vi "messaging_processor.vi"(2 "params":T1={"hla_adapter_port"=2222, "hla_adapter_ip"="", "listener_port"=2222}, 4 "is_simulation_mode":bool=TRUE) -> ()   [LabVIEW 2016]
uses:
  controls/messaging_processor_params.ctl
  controls/messaging_processor_actions.ctl
  controls/terminal_display_handler_actions.ctl
  controls/queue_assistant_actions.ctl
  controls/queue_type.ctl
  controls/event_assistant_actions.ctl
  controls/user_event_item.ctl
  controls/user_events.ctl
panel:
  in  "stop":bool
  in  "reset":bool
  in  "classpaths":string[](array[string])
  in  "exit":bool
  out "out_conn":bool
  out "in_conn":bool
  out "to_hla_history":string
  out "from_hla_history":string
  out "error out":errorcluster
  in  "error in (no error)":errorcluster
  # "Incoming From HLA"
  # "Outgoing To HLA"
  # "connected"
  # "connected"
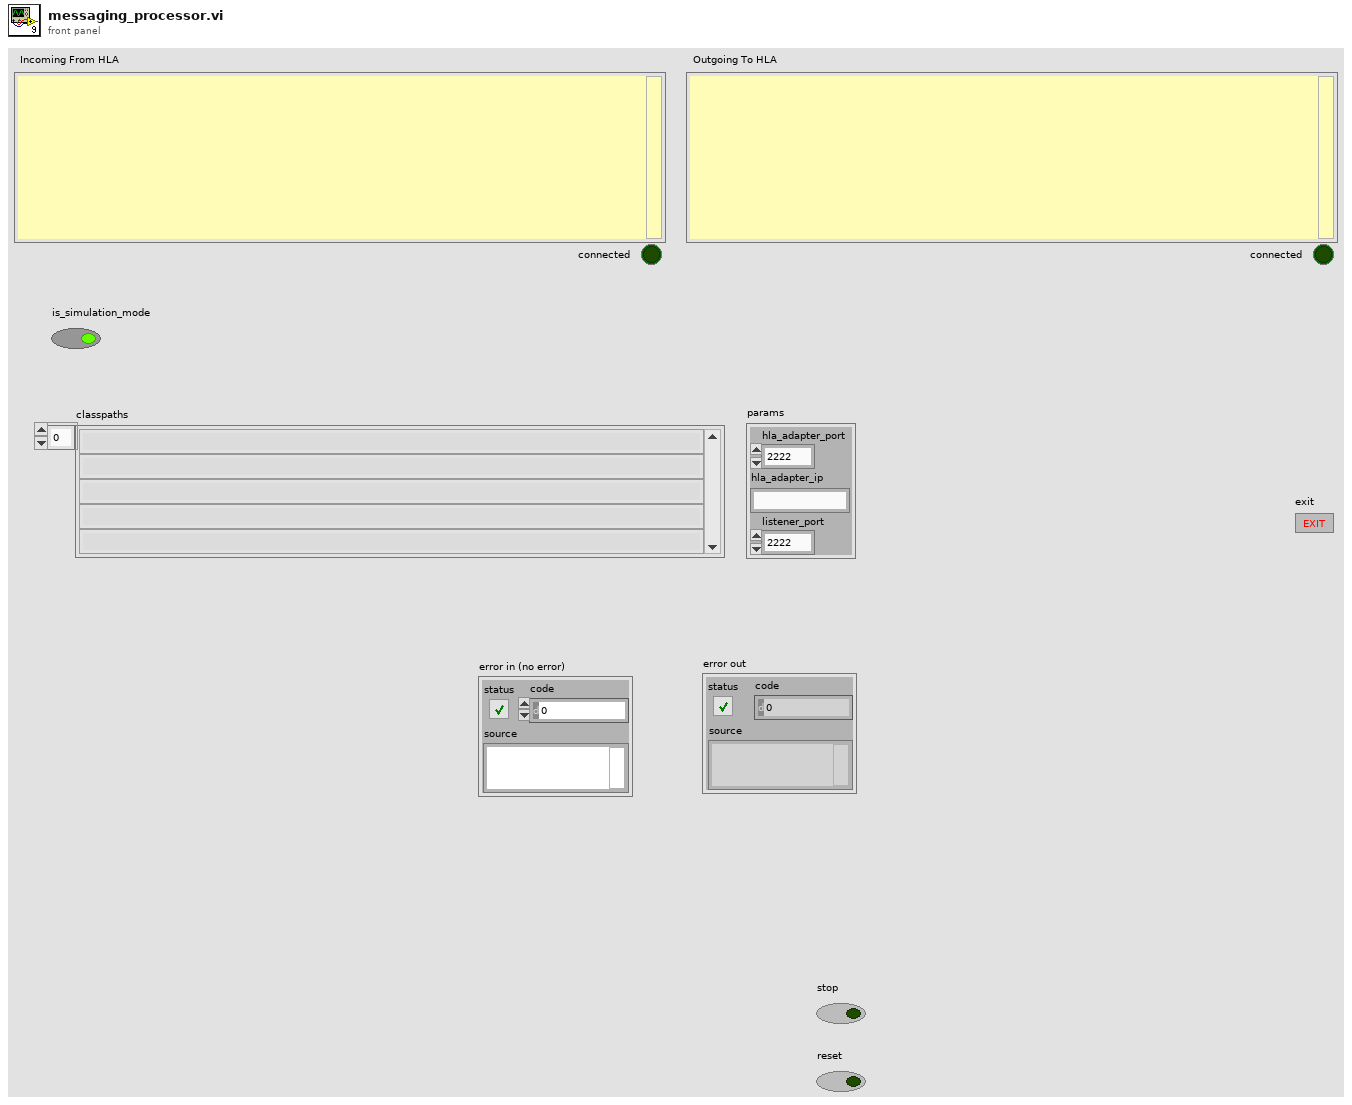
[diagram p1: front panel]
types:
  T1 = typedef "messaging_processor_params.ctl" = cluster{"hla_adapter_port":u16, "hla_adapter_ip":string, "listener_port":u16}
  T2 = typedef "messaging_processor_actions.ctl" = enum16{"-------- unused --------", "establish_connections", "exit", "init", "init_ui", "process_events"}
  T3 = typedef "terminal_display_handler_actions.ctl" = enum16{"clear", "clear_all", "init", "reset", "write"}
  T4 = typedef "queue_assistant_actions.ctl" = enum16{"--- unused ---", "bulk_enq_ahead", "bulk_enq_behind", "destroy", "empty?", "enq_ahead", "enq_behind", "flush", "get_queues", "init"}
  T5 = typedef "queue_references.ctl" = cluster{"entities_in":refnum<queue>, "entities_out":refnum<queue>, "timestep":refnum<queue>, "response":refnum<queue>}
  T6 = typedef "response.ctl" = cluster{"respType":T7, "flattenedContent":string}
  T7 = typedef "response_type.ctl" = string
  T8 = enum16{"Standard", "Buffered", "CRLF", "Immediate"}
  T9 = typedef "queue_type.ctl" = enum16{"all", "dostep", "entities_incoming", "entities_outoing", "response"}
  T10 = typedef "user_event_item.ctl" = cluster{"event":T11, "data":variant}
  T11 = typedef "user_events.ctl" = enum16{"abort", "do-step", "sim-end"}
  T12 = typedef "event_assistant_actions.ctl" = enum16{"--- unused ---", "destroy", "fire", "get_ref", "init"}
  T13 = typedef "lineitem_types.ctl" = enum16{"<unknown>", "received.dostep", "received.item", "received.simend"}
  T14 = typedef "entity.ctl" = cluster{"type":T15, "classPath":string, "params":string[][], "instanceName":string}
  T15 = typedef "entity_type.ctl" = string
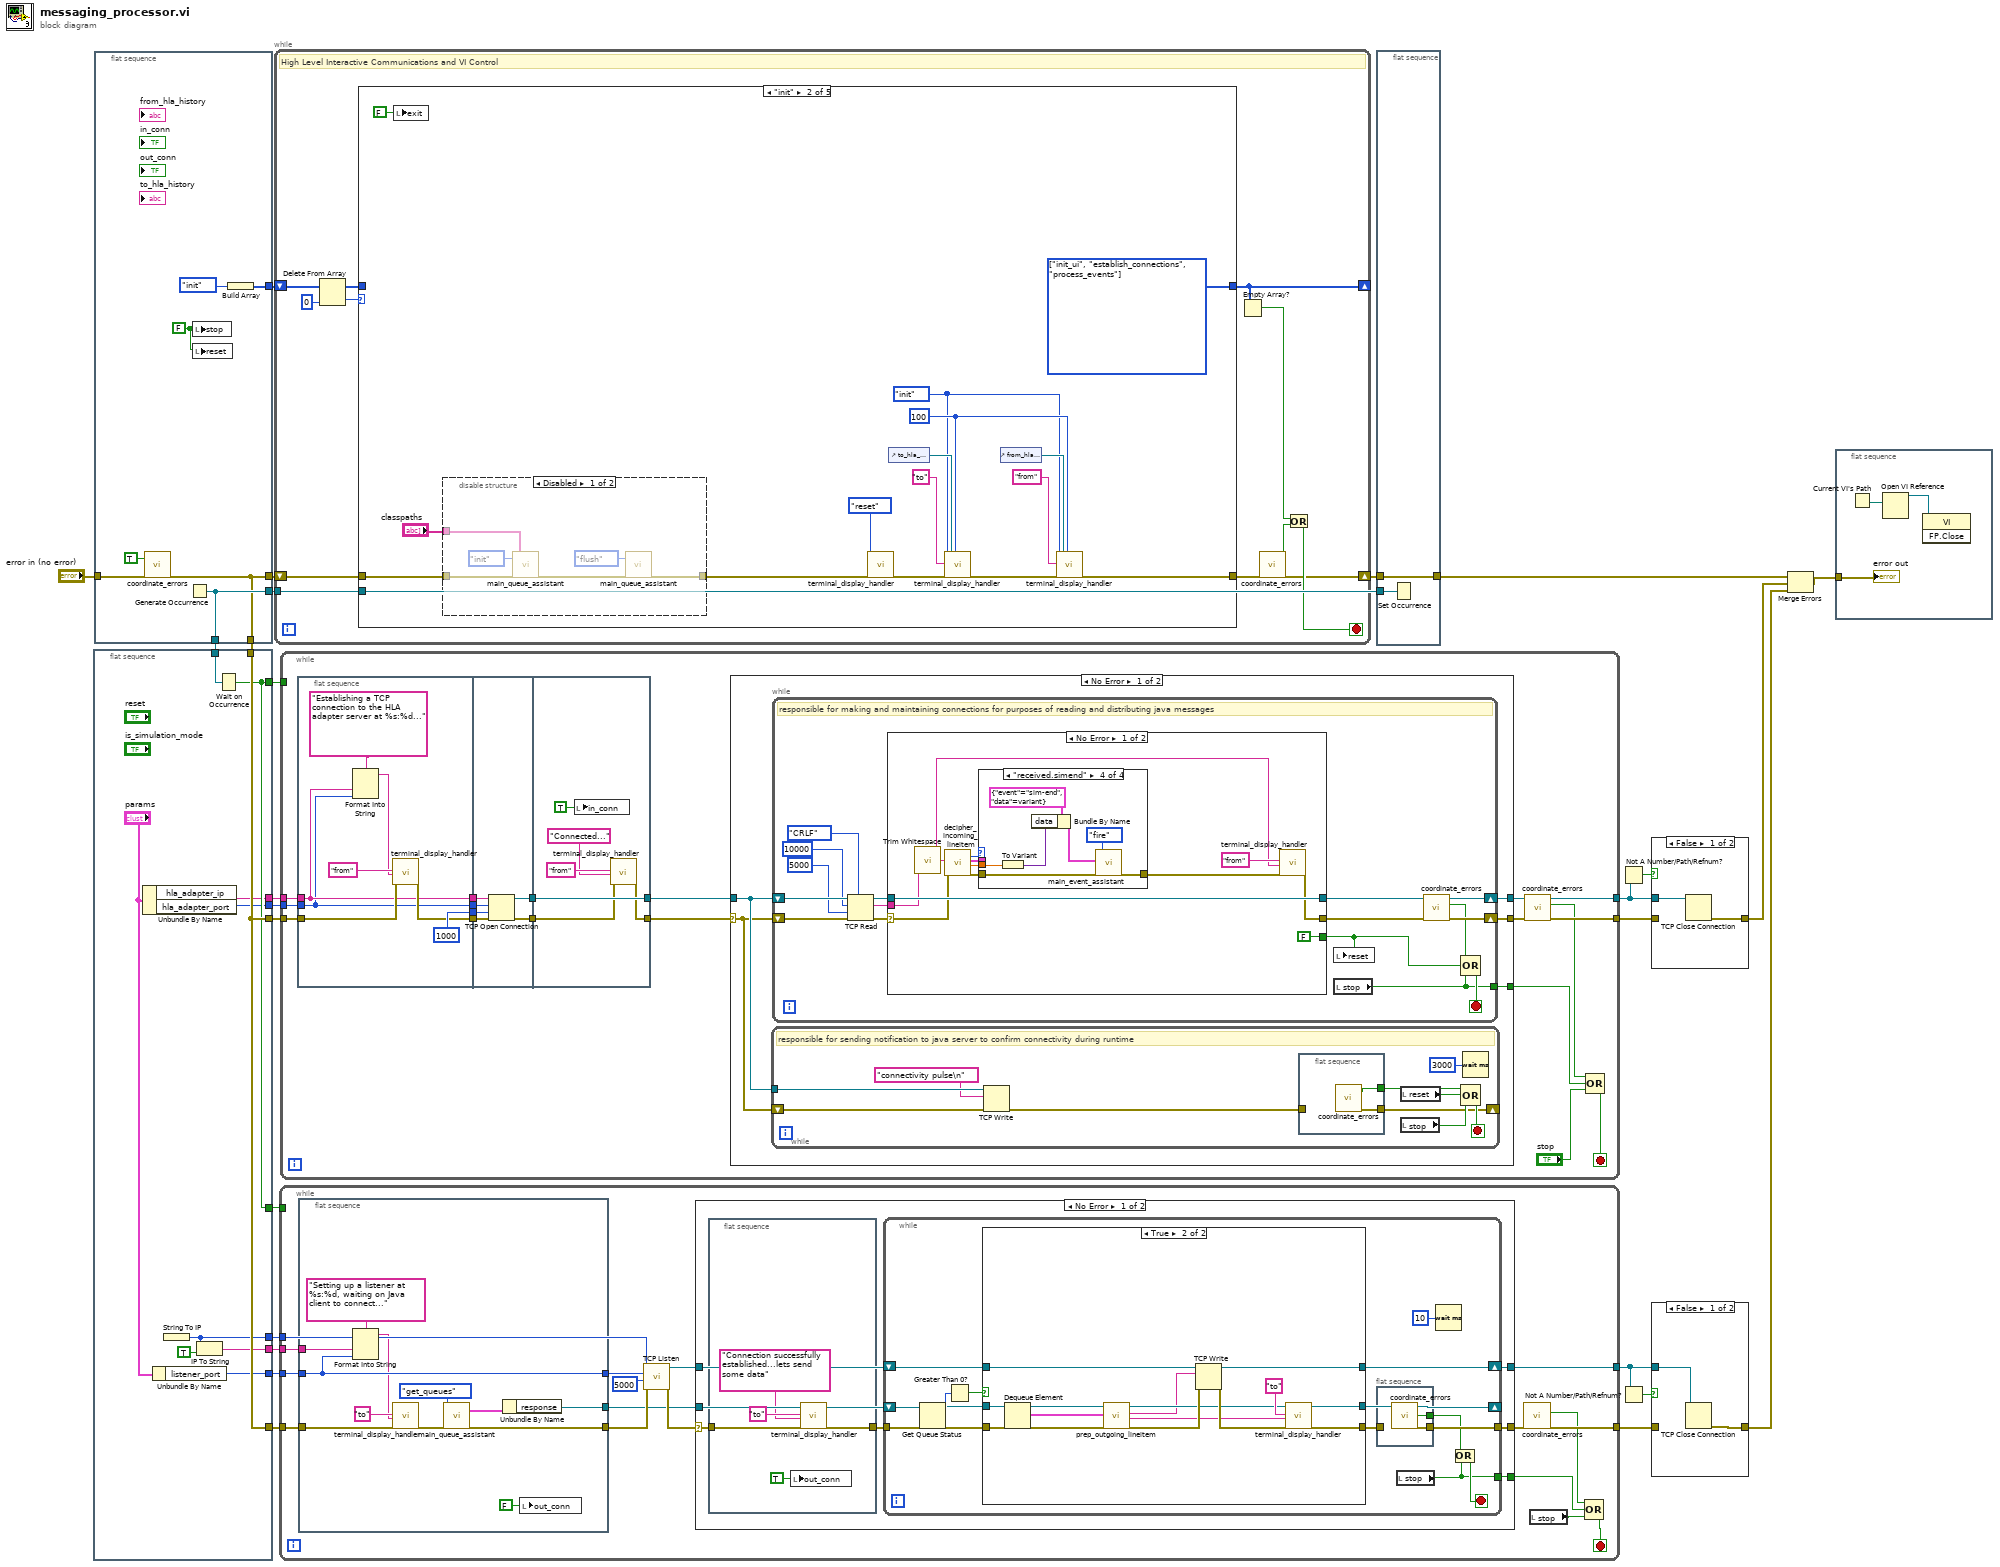
[diagram p0: block diagram]
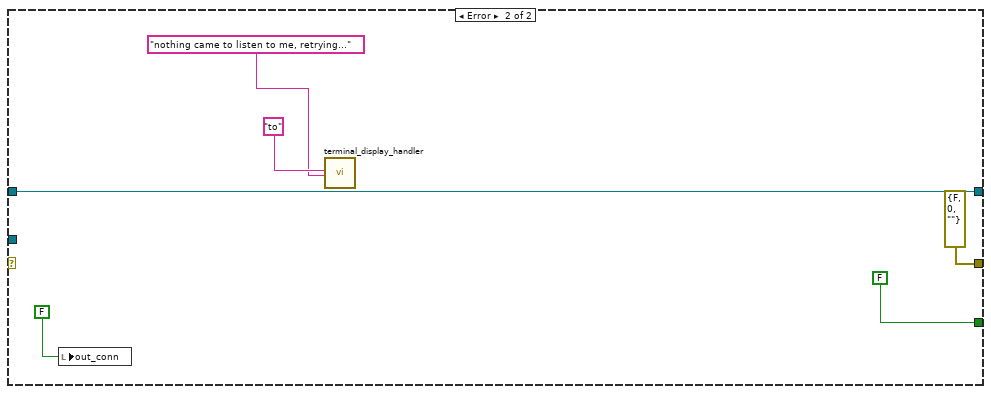
[diagram p5: hidden frame]
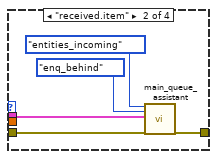
[diagram p7: hidden frame]
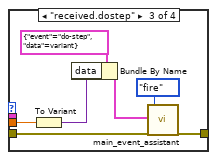
[diagram p8: hidden frame]
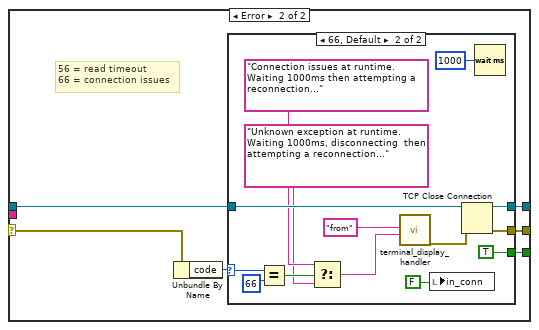
[diagram p9: hidden frame]
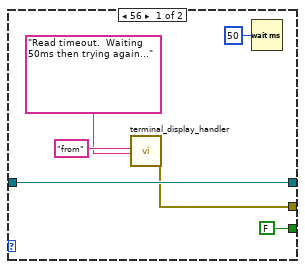
[diagram p10: hidden frame]
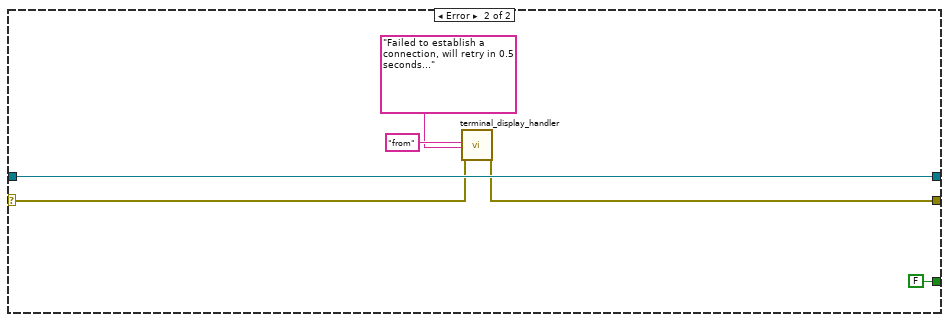
[diagram p11: hidden frame]
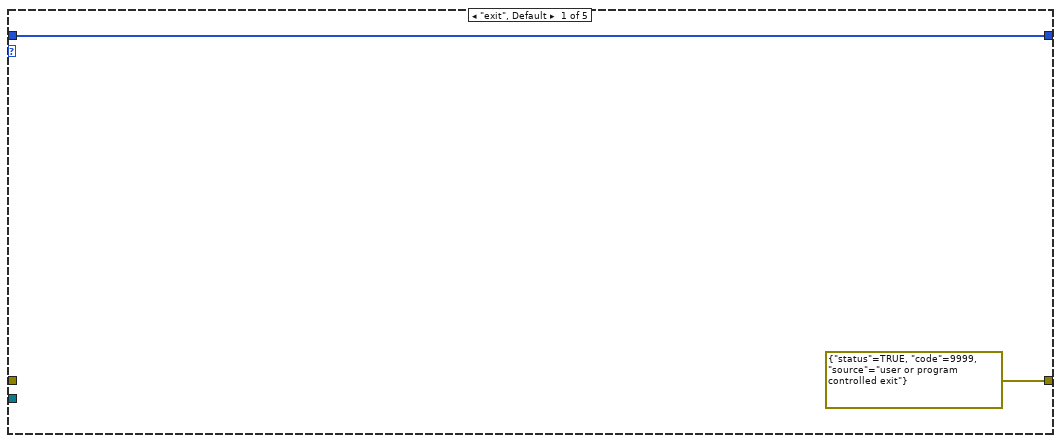
[diagram p12: hidden frame]
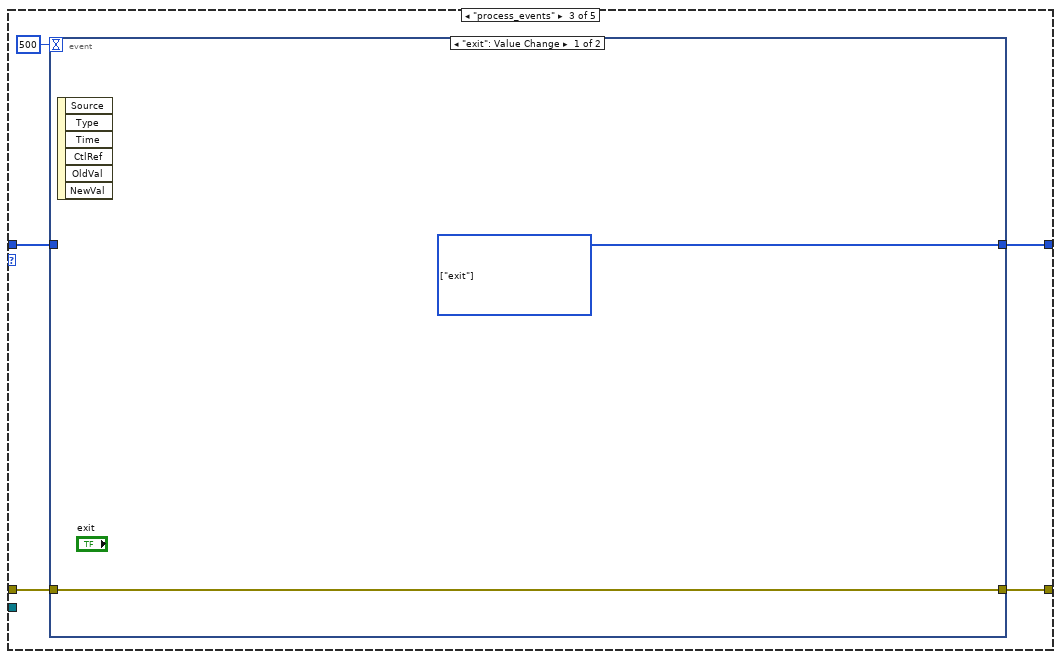
[diagram p14: hidden frame]
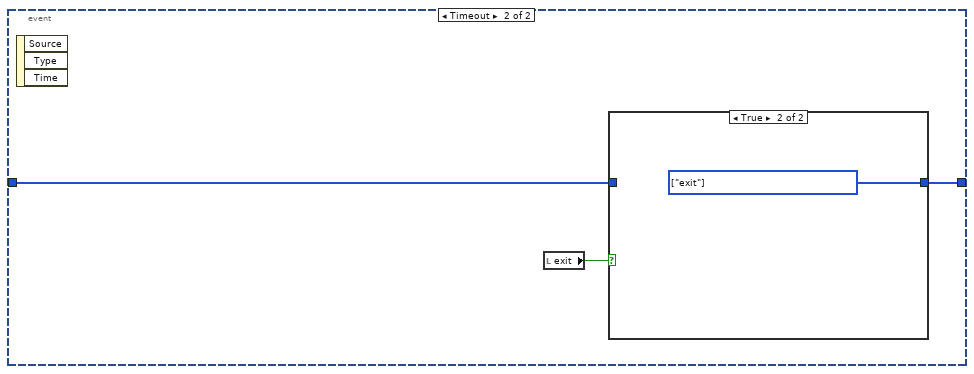
[diagram p15: hidden frame]
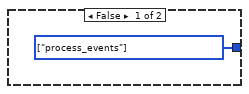
[diagram p16: hidden frame]
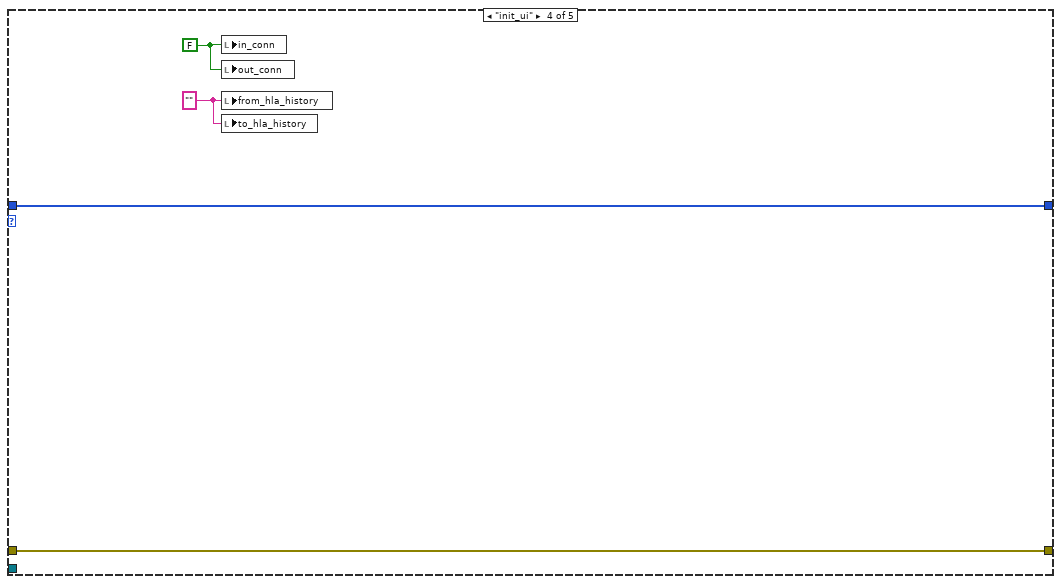
[diagram p17: hidden frame]
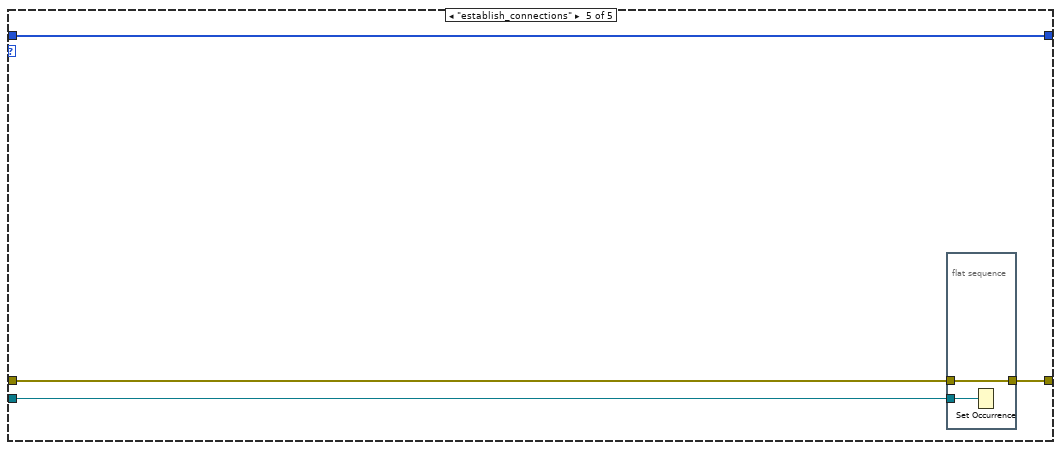
[diagram p18: hidden frame]
diagram:
  n1 = flat-sequence {
    tunnel: w23 -> [w36]
    tunnel: [w36] -> w12
    tunnel: [w36] -> w8
    tunnel: w22 -> [w35]
    tunnel: [w34] -> w5
    tunnel: [w34] -> w4
    tunnel: [w33] -> w11
    tunnel: [w32] -> w10
    tunnel: [w30] -> w9
    tunnel: [w28] -> w3
    tunnel: [w27] -> w2
    frame #0 {
      n2 = Unbundle By Name("params") -> ("hla_adapter_ip"=w33:string, "hla_adapter_port"=w32:u16)
      n3 = Unbundle By Name("params") -> ("listener_port"=w30:u16)
      n4 = String To IP() -> (0:w27:u32)  [unwired: 1 in]
      n5 = IP To String(1:TRUE ("dot notation? (F)"), 2:w27) -> (0:w28:string)
      n6 = Wait on Occurrence(2:w35) -> (0:w34:bool)  [unwired: 2 in]
    }
  }
  n7 = flat-sequence {
    tunnel: [w42] -> w26
    tunnel: "error in (no error)" -> [w41]
    tunnel: [w37] -> w25
    tunnel: [w39] -> w20
    tunnel: [w37] -> w23
    tunnel: [w39] -> w22
    frame #0 {
      w38 = FALSE ("stop")
      n8 = call "coordinate_errors.vi"("reset"=TRUE, "error in (no error)"=w41) -> ("error"=w37:errorcluster)  [unwired: 16 in, 1 out]
      n9 = Generate Occurrence() -> (w39:refnum<k4>)
      n10 = local write "stop"(w38) -> ()
      n11 = local write "reset"(w38) -> ()
      n12 = Build Array(messaging_processor_actions."init" ("actions")) -> (w42:T2[])
    }
  }
  n13 = while {
    shift-right: [w47] -> w21
    shift-left: w25 -> [w52]
    shift-right: [w51] -> _
    shift-left: w26 -> [w55]
    tunnel: w20 -> [w44]
    stop <- w49 stop-if-true
    # "High Level Interactive Communications and VI Control"
    n14 = Delete From Array(array=w55, index=0) -> (deleted portion=w53:T2, array with subset deleted=w45:T2[])  [unwired: 1 in]
    n15 = case shown="\"init\"" w53 {
      tunnel: [w56 w72 w83 w92 w98] -> w51
      tunnel: [errorcluster {"status"=TRUE, "code"=9999, "source"="user or program controlled exit"} ("error") w60 w81 w91 w96] -> w48
      tunnel: w52 -> [_ w71 w82 w91 w97]
      tunnel: w45 -> [w56 _ w79 w92 w98]
      tunnel: w44 -> [_ _ _ _ w95]
      frame "exit", Default {
      }
      frame "init" {
        w66 = 100
        w65 = terminal_display_handler_actions."init" ("actions")
        w72 = T2[] [enum."init_ui", enum."establish_connections", enum."process_events"] items=["-------- unused --------", "establish_connections", "exit", "init", "init_ui", "process_events"]
        n16 = local write "exit"(FALSE ("exit")) -> ()
        n17 = disable-structure shown="Disabled" {
          disable-tunnel: w71 -> [w78 _]
          disable-tunnel: "classpaths" -> [w74 _]
          disable-tunnel: [w73 _] -> w63
          frame Disabled {
            n18 = call "main_queue_assistant.vi"("action (enq_behind = def)"=queue_assistant_actions."init" ("queue_action (enq_behind = def)"), "error in (no error)"=w78, "classpaths_for_queue_identification (ids)"=w74) -> ("error out"=w75:errorcluster)  [unwired: 14 in, 2 out]
            n19 = call "main_queue_assistant.vi"("action (enq_behind = def)"=queue_assistant_actions."flush" ("queue_action (enq_behind = def)"), "error in (no error)"=w75) -> ("error out"=w73:errorcluster)  [unwired: 15 in, 2 out]
          }
          frame Enabled {
          }
        }
        n20 = call "terminal_display_handler.vi"("actions (write=def)"=terminal_display_handler_actions."reset" ("actions"), "error in (no error)"=w63) -> ("error out"=w62:errorcluster)  [unwired: 17 in]
        n21 = control-ref of="to_hla_history"() -> (w68:refnum<vi>)
        n22 = call "terminal_display_handler.vi"("actions (write=def)"=w65, "terminal_name (in)"="to", "error in (no error)"=w62, "terminal_ref (in)"=w68, "buffer (in)"=w66) -> ("error out"=w61:errorcluster)  [unwired: 14 in]
        n23 = control-ref of="from_hla_history"() -> (w67:refnum<vi>)
        n24 = call "terminal_display_handler.vi"("actions (write=def)"=w65, "terminal_name (in)"="from", "error in (no error)"=w61, "terminal_ref (in)"=w67, "buffer (in)"=w66) -> ("error out"=w60:errorcluster)  [unwired: 14 in]
      }
      frame "process_events" {
        n25 = event shown="[0] \"exit\": Value Change" {
          selector: _ -> [_ _]
          dyn-events: _ -> [_ _]
          timeout: 500 -> [_ _]
          tunnel: [w85 w86] -> w83
          tunnel: [w84 _] -> w81
          tunnel: w82 -> [w84 _]
          tunnel: w79 -> [_ w87]
          event "exit": Value Change {
            w85 = T2[] [enum."exit"] items=["-------- unused --------", "establish_connections", "exit", "init", "init_ui", "process_events"]
            n26 = event-data() -> ()  [unwired: 1 in, 6 out]
          }
          event Timeout {
            n27 = event-data() -> ()  [unwired: 1 in, 3 out]
            n28 = local read "exit"() -> (w88:bool)
            n29 = case shown="True" w88 {
              tunnel: w87 -> [_ _]
              tunnel: [w89 w90] -> w86
              frame False {
                w89 = T2[] [enum."process_events"] items=["-------- unused --------", "establish_connections", "exit", "init", "init_ui", "process_events"]
              }
              frame True {
                w90 = T2[] [enum."exit"] items=["-------- unused --------", "establish_connections", "exit", "init", "init_ui", "process_events"]
              }
            }
          }
        }
      }
      frame "init_ui" {
        w93 = "" ("from_hla_history")
        w94 = FALSE ("is_outgoing_connected")
        n30 = local write "in_conn"(w94) -> ()
        n31 = local write "out_conn"(w94) -> ()
        n32 = local write "from_hla_history"(w93) -> ()
        n33 = local write "to_hla_history"(w93) -> ()
      }
      frame "establish_connections" {
        n34 = flat-sequence {
          tunnel: w97 -> [w100]
          tunnel: [w100] -> w96
          tunnel: w95 -> [w99]
          frame #0 {
            n35 = Set Occurrence(w99) -> ()
          }
        }
      }
    }
    n36 = Empty Array?(array=w51) -> (empty?=w50:bool)
    n37 = call "coordinate_errors.vi"("error in (no error)"=w48) -> ("status"=w46:bool, "error"=w47:errorcluster)  [unwired: 17 in]
    n38 = Or(x=w50, y=w46) -> (x .or. y?=w49:bool)
  }
  n39 = while {
    tunnel: w8 -> [w111]
    tunnel: w9 -> [w109]
    tunnel: [w105] -> w1
    tunnel: [w112] -> w17
    tunnel: w4 -> [_]
    tunnel: w3 -> [w102]
    tunnel: w2 -> [w101]
    stop <- w113 stop-if-true
    n40 = flat-sequence {
      tunnel: [w125] -> w110
      tunnel: w111 -> [w129]
      tunnel: [w123] -> w108
      tunnel: w109 -> [w123]
      tunnel: [w119] -> w103
      tunnel: w102 -> [w122]
      frame #0 {
        n41 = Format Into String(format string="Setting up a listener at %s:%d, waiting on Java client to connect..." ("status (d)"), w122, w123) -> (resulting string=w118:string)  [unwired: 2 in, 1 out]
        n42 = call "terminal_display_handler.vi"("terminal_name (in)"="to", "line in"=w118, "error in (no error)"=w129) -> ("error out"=w126:errorcluster)  [unwired: 16 in]
        n43 = call "main_queue_assistant.vi"("action (enq_behind = def)"=queue_assistant_actions."get_queues" ("queue_action (enq_behind = def)"), "error in (no error)"=w126) -> ("refs (out)"=w120:T5, "error out"=w125:errorcluster)  [unwired: 15 in, 1 out]
        n44 = Unbundle By Name(w120) -> ("response"=w119:refnum<queue>)
        n45 = local write "out_conn"(FALSE ("out_conn")) -> ()
      }
    }
    n46 = call <vilib>:"TCP Listen.vi"("net address"=w101, "error in (no error)"=w110, "timeout ms (wait forever: -1)"=5000, "port"=w108) -> ("error out"=w107:errorcluster, "connection ID"=w114:refnum<k5>)  [unwired: 3 in, 3 out]
    n47 = case shown="No Error" w107 {
      selector: w107 -> [w132 _]
      tunnel: [w136 FALSE] -> w115
      tunnel: w114 -> [w135 w179]
      tunnel: [w134 errorcluster {"status"=FALSE, "code"=0, "source"=""} ("error")] -> w106
      tunnel: [w133 w179] -> w112
      tunnel: w103 -> [w130 _]
      frame No Error {
        n48 = flat-sequence {
          tunnel: w132 -> [w139]
          tunnel: [w138] -> w131
          frame #0 {
            n49 = local write "out_conn"(TRUE ("out_conn")) -> ()
            n50 = call "terminal_display_handler.vi"("terminal_name (in)"="to", "line in"="Connection successfully established...lets send some data" ("status (d)"), "error in (no error)"=w139) -> ("error out"=w138:errorcluster)  [unwired: 16 in]
          }
        }
        n51 = while {
          tunnel: [w152] -> w136
          tunnel: w131 -> [w144]
          shift-right: [w154] -> w133
          shift-left: w135 -> [w155]
          tunnel: [w151] -> w134
          shift-right: [w142] -> _
          shift-left: w130 -> [w148]
          stop <- w153 stop-if-true
          n52 = Get Queue Status(queue=w148, error in (no error)=w144) -> (queue out=w145:refnum<queue>, error out=w143:errorcluster, # elements in queue=w147:i32)  [unwired: 1 in, 5 out]
          n53 = Greater Than 0?(x=w147) -> (x > 0?=w146:bool)
          n54 = case shown="True" w146 {
            tunnel: w155 -> [w159 w172]
            tunnel: [w159 w164] -> w154
            tunnel: [w157 w163] -> w149
            tunnel: w143 -> [w157 w166]
            tunnel: w145 -> [w158 w167]
            tunnel: [w158 w165] -> w142
            frame False {
            }
            frame True {
              n55 = Dequeue Element(queue=w167, error in (no error)=w166) -> (queue out=w165:refnum<queue>, element=w162:T6, error out=w168:errorcluster)  [unwired: 1 in, 1 out]
              n56 = call "prep_outgoing_lineitem.vi"("response"=w162, "error in (no error)"=w168) -> ("to_java"=w161:string, "to_terminal"=w160:string, "error out"=w171:errorcluster)  [unwired: 15 in]
              n57 = TCP Write(connection ID=w172, data in=w161, error in (no error)=w171) -> (connection ID out=w164:refnum<k5>, error out=w169:errorcluster)  [unwired: 1 in, 1 out]
              n58 = call "terminal_display_handler.vi"("terminal_name (in)"="to", "line in"=w160, "error in (no error)"=w169) -> ("error out"=w163:errorcluster)  [unwired: 16 in]
            }
          }
          n59 = flat-sequence {
            tunnel: [w174] -> w151
            tunnel: [w173] -> w150
            tunnel: w149 -> [_]
            frame #0 {
              n60 = call "coordinate_errors.vi"() -> ("status"=w173:bool, "error"=w174:errorcluster)  [unwired: 18 in]
            }
          }
          n61 = local read "stop"() -> (w152:bool)
          n62 = Wait (ms)(milliseconds to wait=u32 10) -> ()  [unwired: 1 out]
          n63 = Compound Arithmetic op=OR(w150, w152) -> (w153:bool)
        }
      }
      frame Error {
        n64 = local write "out_conn"(FALSE ("out_conn")) -> ()
        n65 = call "terminal_display_handler.vi"("terminal_name (in)"="to", "line in"="nothing came to listen to me, retrying..." ("status (d)")) -> ()  [unwired: 17 in, 1 out]
      }
    }
    n66 = call "coordinate_errors.vi"("error in (no error)"=w106) -> ("status"=w104:bool, "error"=w105:errorcluster)  [unwired: 17 in]
    n67 = local read "stop"() -> (w116:bool)
    n68 = Compound Arithmetic op=OR(w104, w115, w116) -> (w113:bool)
  }
  n69 = while {
    tunnel: w11 -> [w198]
    tunnel: w10 -> [w197]
    tunnel: [w182] -> w13
    tunnel: [w192] -> w14
    tunnel: w12 -> [w188]
    tunnel: w5 -> [_]
    stop <- w189 stop-if-true
    n70 = flat-sequence {
      tunnel: w197 -> [w200]
      tunnel: w198 -> [w201]
      tunnel: [w201] -> w187
      tunnel: [w200] -> w186
      tunnel: [1000 ("timeout ms (60000)")] -> w185
      tunnel: [w203] -> w184
      tunnel: w188 -> [w204]
      tunnel: w187 -> [w212]
      tunnel: w186 -> [w211]
      tunnel: w185 -> [w208]
      tunnel: [w210] -> w194
      tunnel: [w209] -> w193
      tunnel: w184 -> [w207]
      tunnel: [w214] -> w195
      tunnel: [w218] -> w196
      tunnel: w194 -> [w218]
      tunnel: w193 -> [w215]
      frame #0 {
        n71 = Format Into String(format string="Establishing a TCP connection to the HLA adapter server at %s:%d...", w201, w200) -> (resulting string=w199:string)  [unwired: 2 in, 1 out]
        n72 = call "terminal_display_handler.vi"("terminal_name (in)"="from", "line in"=w199, "error in (no error)"=w204) -> ("error out"=w203:errorcluster)  [unwired: 16 in]
      }
      frame #1 {
        n73 = TCP Open Connection(address=w212, remote port or service name=w211, timeout ms (60000)=w208, error in (no error)=w207) -> (connection ID=w210:refnum<k5>, error out=w209:errorcluster)  [unwired: 1 in]
      }
      frame #2 {
        n74 = local write "in_conn"(TRUE ("in_conn")) -> ()
        n75 = call "terminal_display_handler.vi"("terminal_name (in)"="from", "line in"="Connected...", "error in (no error)"=w215) -> ("error out"=w214:errorcluster)  [unwired: 16 in]
      }
    }
    n76 = case shown="No Error" w195 {
      selector: w195 -> [w219 w310]
      tunnel: w196 -> [w220 w314]
      tunnel: [w223 w309] -> w183
      tunnel: [w222 w314] -> w192
      tunnel: [w221 FALSE ("stop")] -> w190
      frame No Error {
        n77 = while {
          tunnel: w220 -> [w233]
          shift-right: [w226] -> _
          shift-left: w219 -> [w230]
          stop <- w227 stop-if-true
          # "responsible for sending notification to java server to confirm connectivity during runtime"
          n78 = TCP Write(connection ID=w233, data in="connectivity pulse\n", error in (no error)=w230) -> (error out=w224:errorcluster)  [unwired: 1 in, 2 out]
          n79 = flat-sequence {
            tunnel: [w235] -> w226
            tunnel: [w234] -> w225
            tunnel: w224 -> [_]
            frame #0 {
              n80 = call "coordinate_errors.vi"() -> ("status"=w234:bool, "error"=w235:errorcluster)  [unwired: 18 in]
            }
          }
          n81 = local read "reset"() -> (w229:bool)
          n82 = local read "stop"() -> (w228:bool)
          n83 = Compound Arithmetic op=OR(w225, w229, w228) -> (w227:bool)
          n84 = Wait (ms)(milliseconds to wait=u32 3000) -> ()  [unwired: 1 out]
        }
        n85 = while {
          shift-right: [w238] -> w223
          shift-left: w219 -> [w242]
          shift-right: [w249] -> w222
          shift-left: w220 -> [w246]
          tunnel: [w247] -> w221
          stop <- w248 stop-if-true
          # "responsible for making and maintaining connections for purposes of reading and distributing java messages"
          n86 = TCP Read(connection ID=w246, bytes to read=10000, error in (no error)=w242, 7:T8."CRLF" ("mode (standard)"), 9:5000 ("timeout ms (25000)")) -> (connection ID out=w241:refnum<k5>, data out=w236:string, error out=w250:errorcluster)
          n87 = case shown="No Error" w250 {
            selector: w250 -> [w256 w284]
            tunnel: [w261 w287] -> w249
            tunnel: w241 -> [w261 w288]
            tunnel: [w255 w286] -> w239
            tunnel: [FALSE w285] -> w240
            tunnel: w236 -> [w260 _]
            frame No Error {
              n88 = call <vilib>:"Trim Whitespace.vi"("string"=w260) -> ("trimmed string"=w252:string)  [unwired: 1 in]
              n89 = call "decipher_incoming_lineitem.vi"("lineitem (in)"=w252, "error in (no error)"=w256) -> ("lineitem_type (out)"=w254:T13, "clustered_item (out)"=w258:T14, "timestep (out)"=w253:dbl, "error out"=w259:errorcluster)  [unwired: 14 in]
              n90 = case shown="\"received.simend\"" w254 {
                tunnel: w259 -> [w263 w266 w275 w282]
                tunnel: w258 -> [_ w265 _ _]
                tunnel: [w263 w264 w274 w281] -> w251
                tunnel: w253 -> [_ _ w271 w278]
                frame Default {
                }
                frame "received.item" {
                  n91 = call "main_queue_assistant.vi"("queue_type (def=all)"=queue_type."entities_incoming" ("queue_type (def=both)"), "action (enq_behind = def)"=queue_assistant_actions."enq_behind" ("queue_action (enq_behind = def)"), "entity"=w265, "error in (no error)"=w266) -> ("error out"=w264:errorcluster)  [unwired: 13 in, 2 out]
                }
                frame "received.dostep" {
                  n92 = To Variant(anything=w271) -> (Variant=w269:variant)
                  n93 = Bundle By Name(cluster=T10 {"event"=enum."do-step", "data"=variant} ("event_item"), "data"=w269) -> (w270:T10)
                  n94 = call "main_event_assistant.vi"("event_action (enq_behind = def)"=event_assistant_actions."fire", "event_item (in)"=w270, "error in (no error)"=w275) -> ("error out"=w274:errorcluster)  [unwired: 15 in, 1 out]
                }
                frame "received.simend" {
                  n95 = To Variant(anything=w278) -> (Variant=w276:variant)
                  n96 = Bundle By Name(cluster=T10 {"event"=enum."sim-end", "data"=variant} ("event_item"), "data"=w276) -> (w277:T10)
                  n97 = call "main_event_assistant.vi"("event_action (enq_behind = def)"=event_assistant_actions."fire", "event_item (in)"=w277, "error in (no error)"=w282) -> ("error out"=w281:errorcluster)  [unwired: 15 in, 1 out]
                }
              }
              n98 = call "terminal_display_handler.vi"("terminal_name (in)"="from", "line in"=w252, "error in (no error)"=w251) -> ("error out"=w255:errorcluster)  [unwired: 16 in]
            }
            frame Error {
              # "56 = read timeout\n66 = connection issues"
              n99 = Unbundle By Name(w284) -> ("code"=w283:i32)
              n100 = case shown="66, Default" w283 {
                selector: w283 -> [_ w303]
                tunnel: w288 -> [w292 w306]
                tunnel: [w292 w305] -> w287
                tunnel: [w289 w304] -> w286
                tunnel: [FALSE TRUE] -> w285
                frame 56 {
                  n101 = call "terminal_display_handler.vi"("terminal_name (in)"="from", "line in"="Read timeout.  Waiting 50ms then trying again...") -> ("error out"=w289:errorcluster)  [unwired: 17 in]
                  n102 = Wait (ms)(milliseconds to wait=u32 50) -> ()  [unwired: 1 out]
                }
                frame 66, Default {
                  n103 = Equal?(x=w303, y=66) -> (x = y?=w301:bool)
                  n104 = Select(t="Connection issues at runtime.  Waiting 1000ms then attempting a reconnection...", s=w301, f="Unknown exception at runtime.  Waiting 1000ms, disconnecting  then attempting a reconnection...") -> (s? t:f=w297:string)
                  n105 = call "terminal_display_handler.vi"("terminal_name (in)"="from", "line in"=w297) -> ("error out"=w296:errorcluster)  [unwired: 17 in]
                  n106 = local write "in_conn"(FALSE ("in_conn")) -> ()
                  n107 = TCP Close Connection(connection ID=w306, error in (no error)=w296) -> (connection ID out=w305:refnum<k5>, error out=w304:errorcluster)  [unwired: 1 in]
                  n108 = Wait (ms)(milliseconds to wait=u32 1000) -> ()  [unwired: 1 out]
                }
              }
            }
          }
          n109 = local write "reset"(w240) -> ()
          n110 = local read "stop"() -> (w247:bool)
          n111 = call "coordinate_errors.vi"("error in (no error)"=w239) -> ("status"=w237:bool, "error"=w238:errorcluster)  [unwired: 17 in]
          n112 = Compound Arithmetic op=OR(w237, w240, w247) -> (w248:bool)
        }
      }
      frame Error {
        n113 = call "terminal_display_handler.vi"("terminal_name (in)"="from", "line in"="Failed to establish a connection, will retry in 0.5 seconds...", "error in (no error)"=w310) -> ("error out"=w309:errorcluster)  [unwired: 16 in]
      }
    }
    n114 = call "coordinate_errors.vi"("error in (no error)"=w183) -> ("status"=w181:bool, "error"=w182:errorcluster)  [unwired: 17 in]
    n115 = Compound Arithmetic op=OR(w181, w190, "stop") -> (w189:bool)
  }
  n116 = flat-sequence {
    tunnel: w21 -> [w315]
    tunnel: w20 -> [w316]
    tunnel: [w315] -> w19
    frame #0 {
      n117 = Set Occurrence(w316) -> ()
    }
  }
  n118 = Not A Number/Path/Refnum?(number/path/refnum=w14) -> (NaN/Path/Refnum?=w15:bool)
  n119 = Not A Number/Path/Refnum?(number/path/refnum=w17) -> (NaN/Path/Refnum?=w16:bool)
  n120 = case shown="False" w15 {
    tunnel: w13 -> [_ w319]
    tunnel: [w318 w319] -> w7
    tunnel: w14 -> [w317 _]
    frame False {
      n121 = TCP Close Connection(connection ID=w317) -> (error out=w318:errorcluster)  [unwired: 2 in, 1 out]
    }
    frame True {
    }
  }
  n122 = case shown="False" w16 {
    tunnel: w1 -> [_ w322]
    tunnel: [w321 w322] -> w6
    tunnel: w17 -> [w320 _]
    frame False {
      n123 = TCP Close Connection(connection ID=w320) -> (error out=w321:errorcluster)  [unwired: 2 in, 1 out]
    }
    frame True {
    }
  }
  n124 = Merge Errors(w19, w7, w6) -> (w18:errorcluster)
  n125 = flat-sequence {
    tunnel: w18 -> [w325]
    frame #0 {
      n126 = Current VI's Path() -> (path=w324:path)
      n127 = Open VI Reference(vi path=w324) -> (vi reference=w323:refnum<vi>)  [unwired: 5 in, 1 out]
      n128 = invoke class="VI" method="FP.Close"(reference=w323) -> ()  [unwired: 2 in, 3 out]
      "error out" <- w325
    }
  }
